vi "get channels.vi"(11 "SystemLin Tag Module configuration in":refnum<class "SystemLink File configuration.lvclass">) -> (2 "channels":refnum<class "TBM channel.lvclass">[](array[class]), 3 "SystemLin Tag Module configuration out":refnum<class "SystemLink File configuration.lvclass">)   [LabVIEW 2015, in "SystemLink File configuration.lvclass"]
doc: "Returns an array of all Channels currently added to this configuration object."
uses:
  SystemLink File configuration.lvclass
  <vilib>/NI/Tag Bus Module Framework/channel/TBM channel.lvclass
  SystemLink File configuration.lvclass/SystemLink File configuration.ctl
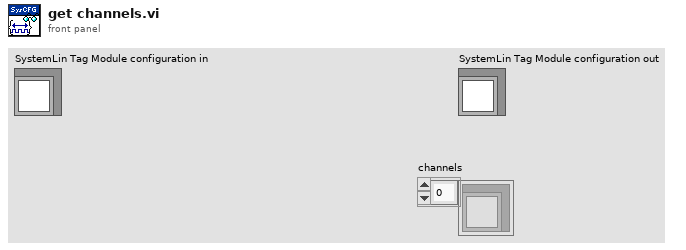
[diagram p1: front panel]
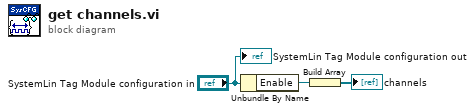
[diagram p0: block diagram]
diagram:
  n1 = Unbundle By Name("SystemLin Tag Module configuration in") -> ("Enable"=w2:refnum<class "TBM channel.lvclass">)
  n2 = Build Array(w2) -> (→"channels":refnum<class "TBM channel.lvclass">[])
  "SystemLin Tag Module configuration out" <- "SystemLin Tag Module configuration in"
